vi "CODMn通讯.vi"() -> ()   [LabVIEW 2016, in "斯坦道CODMn新电路板.lvlib"]
uses:
  <vilib>/NI/Modbus Library/API/Wrapper/Create TCP Slave.vi
  <vilib>/Utility/config.llb/Write Key (String).vi
  <vilib>/Plasmionique/MB Master/MB_Master/MB_Master.lvclass
  <vilib>/NI/Modbus Library/API/slave/Modbus Slave.lvclass
  <vilib>/Utility/config.llb/NI_LVConfig.lvlib
  <vilib>/Plasmionique/MB Master/MB Master.lvlib
  <vilib>/NI/Modbus Library/API/Wrapper/API Main.lvlib
panel:
  out "控制命令 2":u16[](array[numeric]) format="%xH"
  out "状态告警区":T1 {"工作状态" items=["空闲"=0, "水样测试"=1, "标样核查"=2, "零点核查"=3, "跨度核查"=4, "空白测试"=5, "平行样测试"=6, "加标回收"=7, "空白校准"=8, "标样校准"=9, "初始化（清洗）"=10, "调试"=22, "填充管路"=30, "清洗管路"=31, "清洗反应杯"=32]; "告警代码" items=["无告警", "缺试剂告警", "缺水样告警", "缺蒸馏水告警", "缺标液告警", "仪表漏液告警", "标定异常告警", "超量程告警", "加热异常", "低试剂预警", "超上限告警", "超下限告警", "仪表内部其他异常", "滴定异常告警", "电极异常告警", "量程切换告警", "参数设置告警", "PH电极电位异常", "电导率电极异常", "浊度光度异常", "溶解氧电极异常", "溶解氧光强异常", "温度异常告警", "PH异常告警", "溶解氧异常告警", "电导率异常告警", "浊度异常告警", "叶绿素异常告警", "藻密度异常告警", "蓝绿藻异常告警", "ORP异常告警", "氨氮异常告警", "清洁刷异常告警", "SD卡异常告警", "蓝牙异常告警", "Wifi异常告警", "流程异常告警"]; "故障代码" items=["无故障", "电机故障", "温度故障", "通讯故障", "滴定故障"]}
  out "测量数据区":T2 {"单位" items=["ug/L", "mg/L", "ppm", "mg/m3", "cm", "ppb", "ug/m3", "%", "nmol/mol", "umol/mol", "MPN/L", "MPN/100ml", "ng/m3", "NTU", "无量纲", "ms/cm", "us/cm", "℃", "mV", "万个/L"]}
  out "状态告警区":u16[](array[numeric])
  out "测量数据区":u16[](array[numeric])
  out "序列号":string
  out "status":bool
  out "关键参数区":T3
  in  "读关键参数区":bool
  in  "读状态告警区":bool
  in  "读测量数据区":bool
  in  "站号":u16(ring) items=["CODMn"=21, "氨氮"=3]
  in  "停止":bool
  in  "启动":bool
  in  "控制命令":u16(ring) items=["启动测量"=1, "标样核查"=2, "零点核查"=3, "跨度核查"=4, "空白测试"=5, "平行样测试"=6, "加标回收"=7, "空白校准"=8, "标样校准"=9, "初始化（清洗）"=10, "停止测试"=11, "仪器重启"=12, "校时"=13, "模式设置"=14, "测量间隔设置"=15]
  in  "控制命令参数":u16[](array[numeric]) format="%04xH"
  in  "VISA Resource":refnum<visa-resource-name>
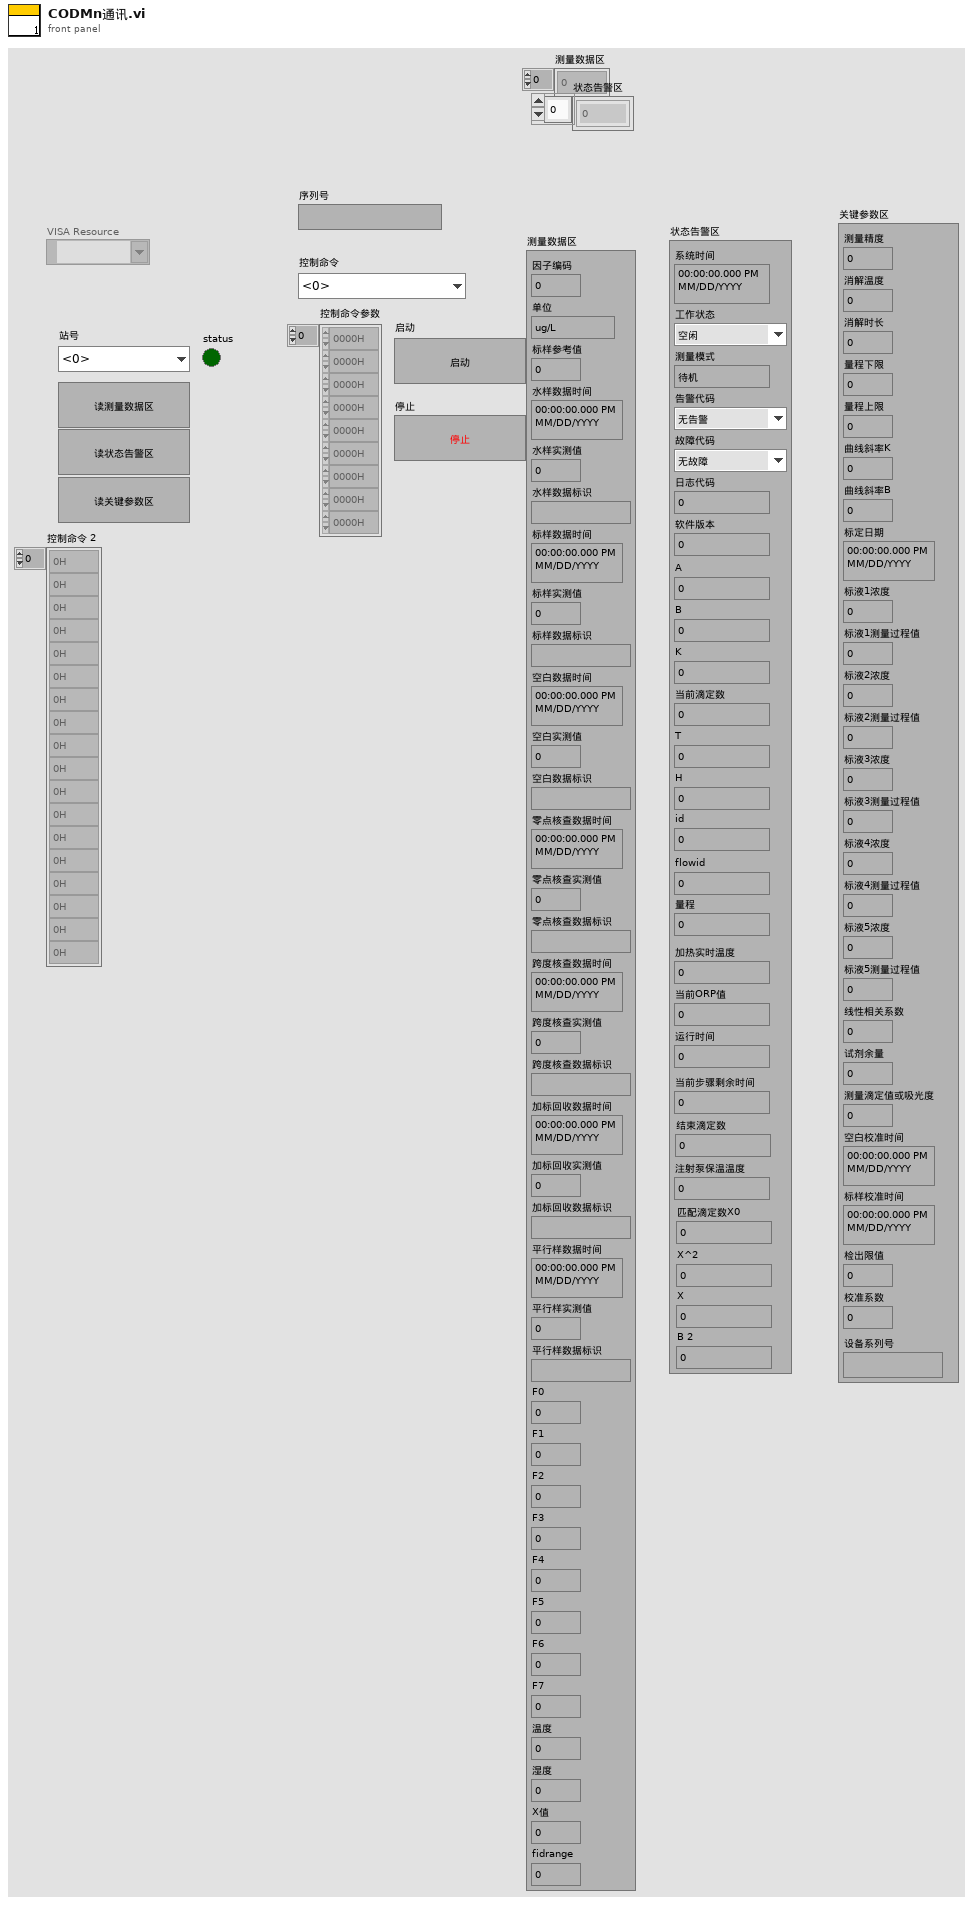
[diagram p1: front panel]
types:
  T1 = cluster{"系统时间":timestamp, "工作状态":u16, "测量模式":enum16{"待机", "连续模式", "周期模式", "定点模式", "受控模式", "手动模式"}, "告警代码":u16, "故障代码":u16, "日志代码":u16, "软件版本":u16, "A":sgl, "B":sgl, "K":sgl, "当前滴定数":sgl, "T":sgl, "H":sgl, "id":u16, "flowid":u16, "量程":u16, "加热实时温度":sgl, "当前ORP值":sgl, "运行时间":sgl, "当前步骤剩余时间":sgl, "结束滴定数":sgl, "注射泵保温温度":sgl, "匹配滴定数X0":u16, "X^2":sgl, "X":sgl, "B 2":sgl}
  T2 = cluster{"因子编码":u32, "单位":u16, "标样参考值":sgl, "水样数据时间":timestamp, "水样实测值":sgl, "水样数据标识":string, "标样数据时间":timestamp, "标样实测值":sgl, "标样数据标识":string, "空白数据时间":timestamp, "空白实测值":sgl, "空白数据标识":string, "零点核查数据时间":timestamp, "零点核查实测值":sgl, "零点核查数据标识":string, "跨度核查数据时间":timestamp, "跨度核查实测值":sgl, "跨度核查数据标识":string, "加标回收数据时间":timestamp, "加标回收实测值":sgl, "加标回收数据标识":string, "平行样数据时间":timestamp, "平行样实测值":sgl, "平行样数据标识":string, "F0":sgl, "F1":sgl, "F2":sgl, "F3":sgl, "F4":sgl, "F5":sgl, "F6":sgl, "F7":sgl, "温度":sgl, "湿度":sgl, "X值":sgl, "fidrange":sgl}
  T3 = cluster{"测量精度":u16, "消解温度":u16, "消解时长":u16, "量程下限":sgl, "量程上限":sgl, "曲线斜率K":sgl, "曲线斜率B":sgl, "标定日期":timestamp, "标液1浓度":sgl, "标液1测量过程值":sgl, "标液2浓度":sgl, "标液2测量过程值":sgl, "标液3浓度":sgl, "标液3测量过程值":sgl, "标液4浓度":sgl, "标液4测量过程值":sgl, "标液5浓度":sgl, "标液5测量过程值":sgl, "线性相关系数":sgl, "试剂余量":u32, "测量滴定值或吸光度":sgl, "空白校准时间":timestamp, "标样校准时间":timestamp, "检出限值":sgl, "校准系数":sgl, "设备系列号":string}
  T4 = cluster{"测量模式":enum16{"水样测量", "标样核查", "零点核查", "跨度核查", "空白测试", "加标回收", "平行样", "校零", "校标"}}
  T5 = typedef "NI_LVConfig.lvlib/Config Data RefNum.ctl" = refnum<k1>
  T6 = cluster{"站号":u16, "量程切换":enum32{"H", "L", "AUTO"}, "控制命令":u16, "模式设置":enum16{"待机", "连续模式", "周期模式", "定点模式", "受控模式", "手动模式"}, "测量间隔":u16}
  T7 = enum16{"水样测量", "标样核查", "零点核查", "跨度核查", "空白测试", "加标回收", "平行样", "校零", "校标"}
  T8 = enum8{"Enabled", "Disabled", "Disabled and Grayed Out"}
  T9 = typedef "量程选择控件.ctl" = enum32{"L", "H", "AUTO"}
  T10 = cluster{"水样测试量程模式":T9, "标样核查量程模式":T9, "零点核查量程模式":T9, "跨度核查量程模式":T9, "空白测试量程模式":T9, "平行样测试量程模式":T9, "加标回收量程模式":T9, "空白校准量程模式":T9, "标样校准量程模式":T9}
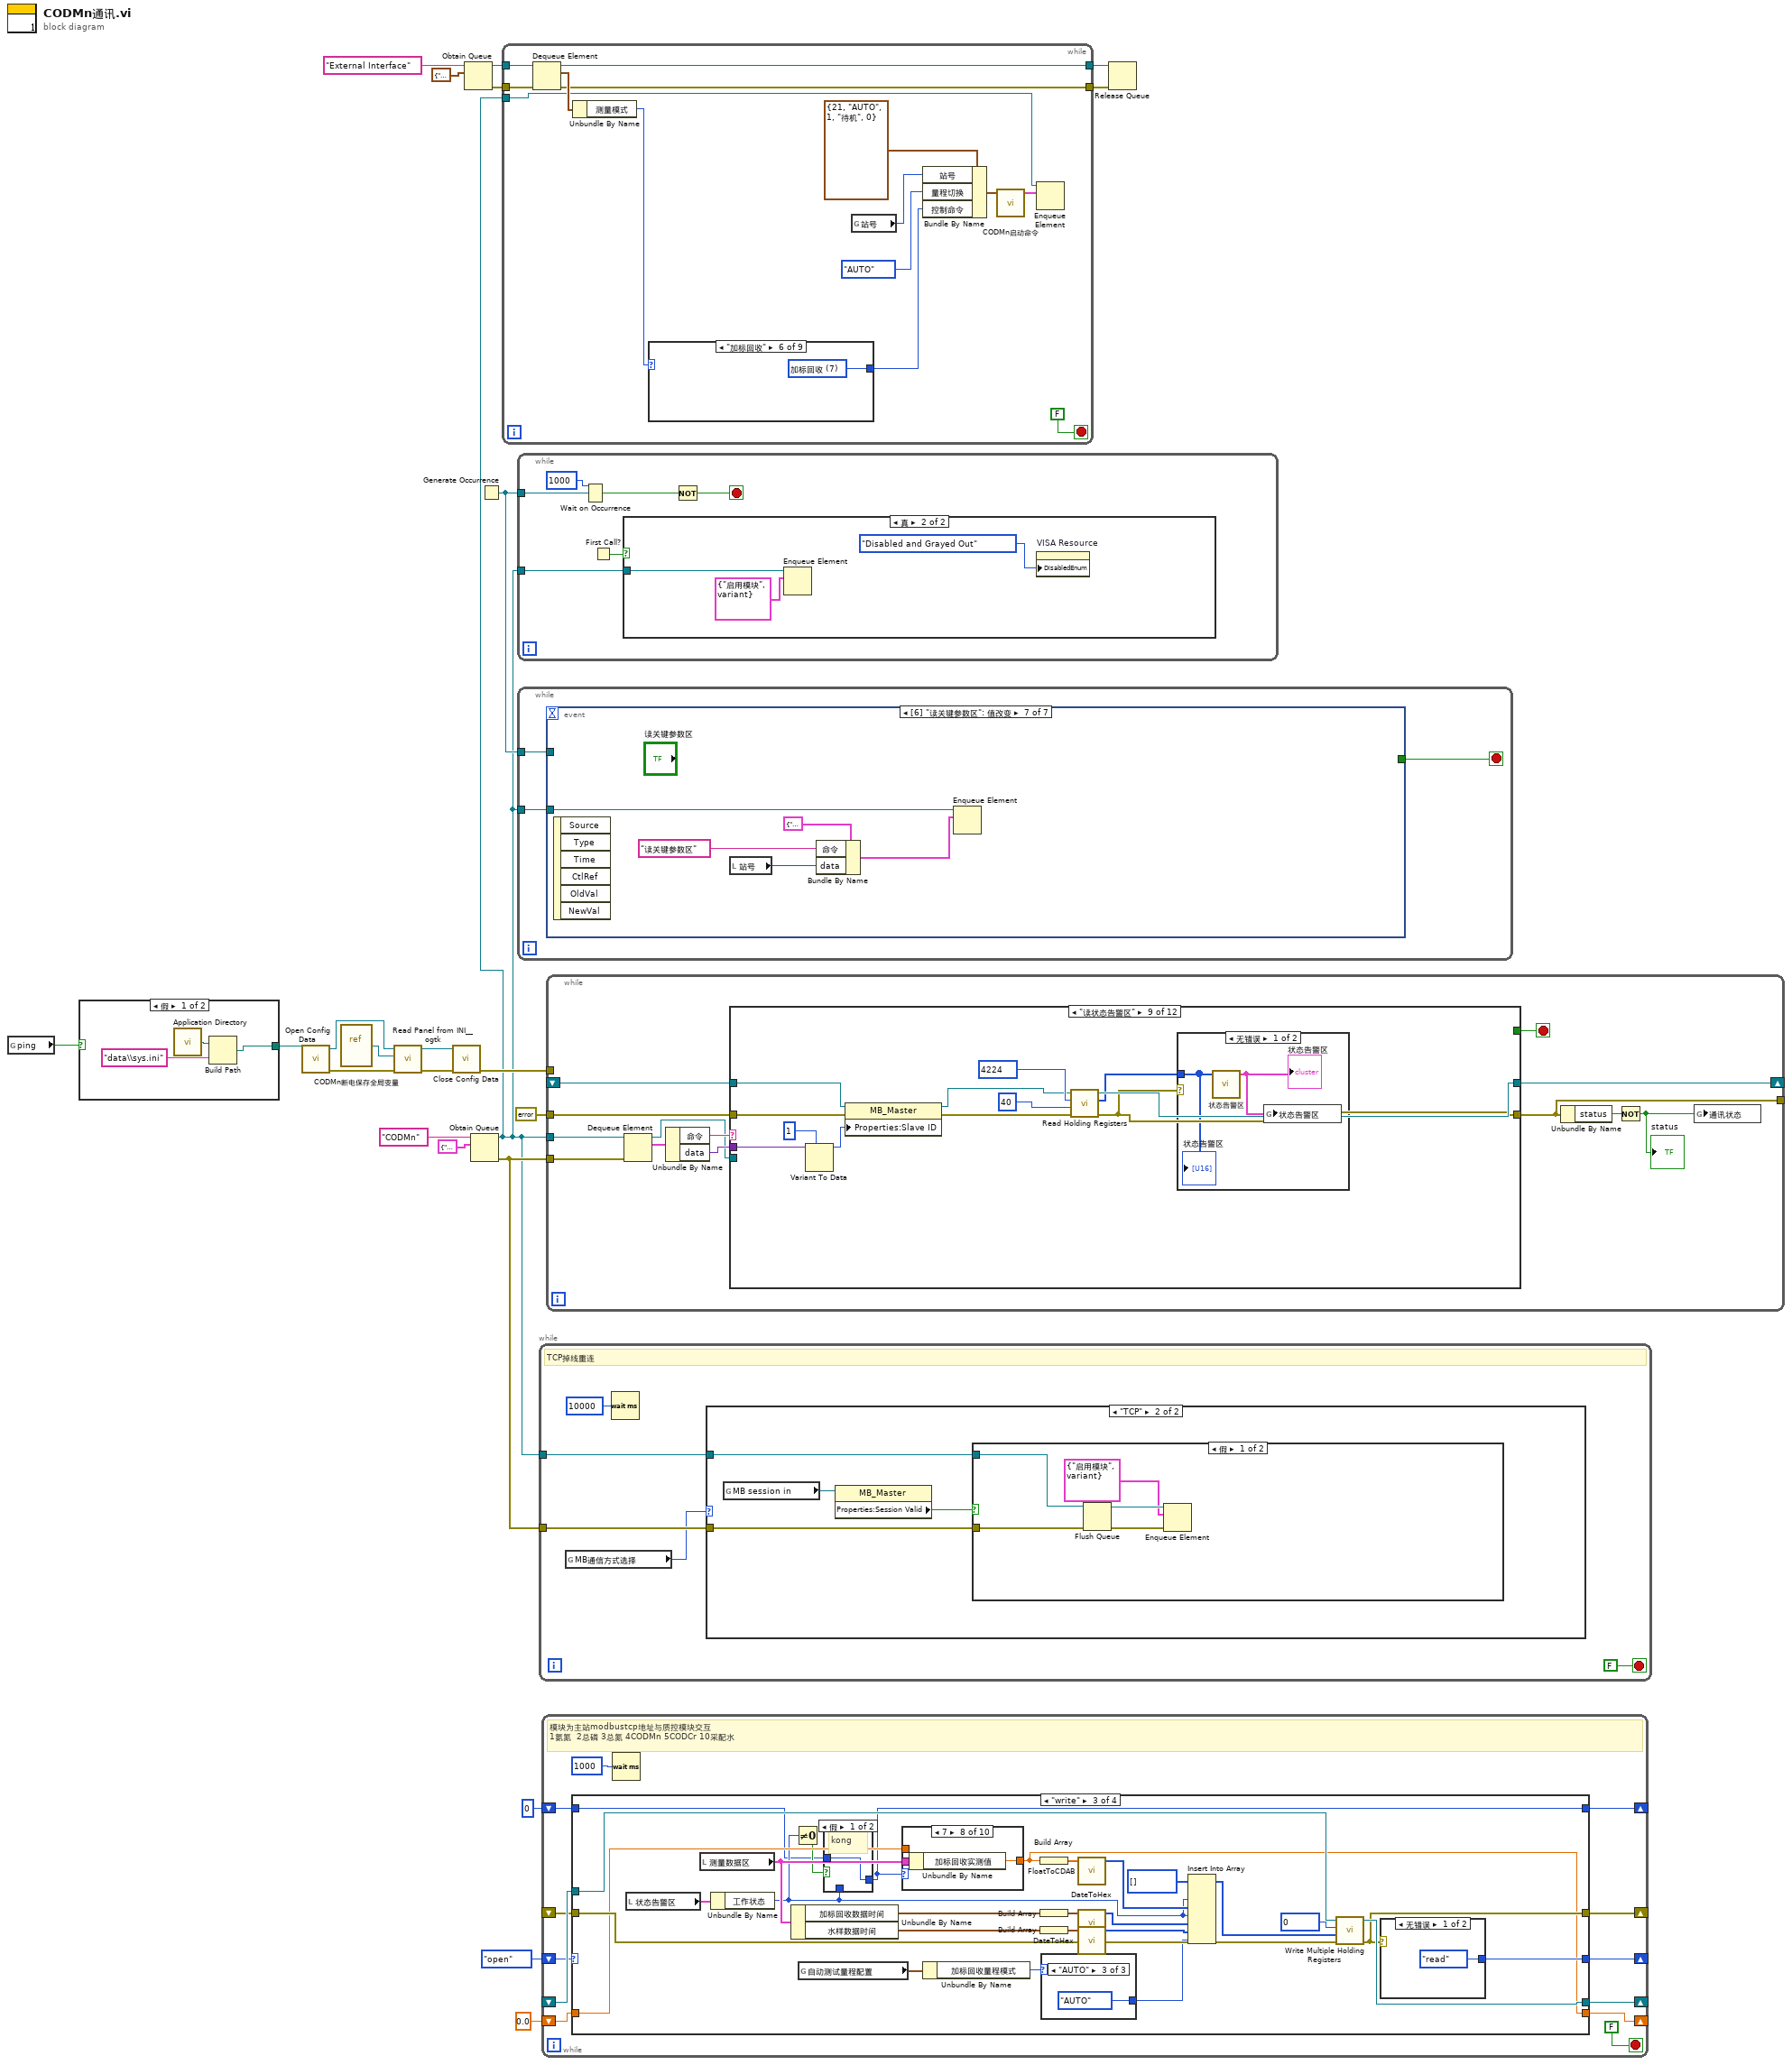
[diagram p0: block diagram]
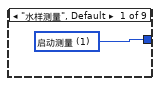
[diagram p2: hidden frame]
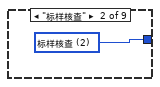
[diagram p3: hidden frame]
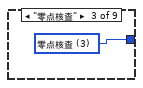
[diagram p4: hidden frame]
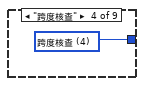
[diagram p5: hidden frame]
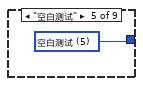
[diagram p6: hidden frame]
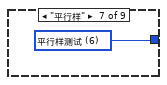
[diagram p7: hidden frame]
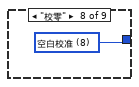
[diagram p8: hidden frame]
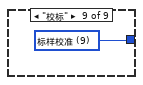
[diagram p9: hidden frame]
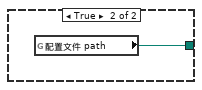
[diagram p10: hidden frame]
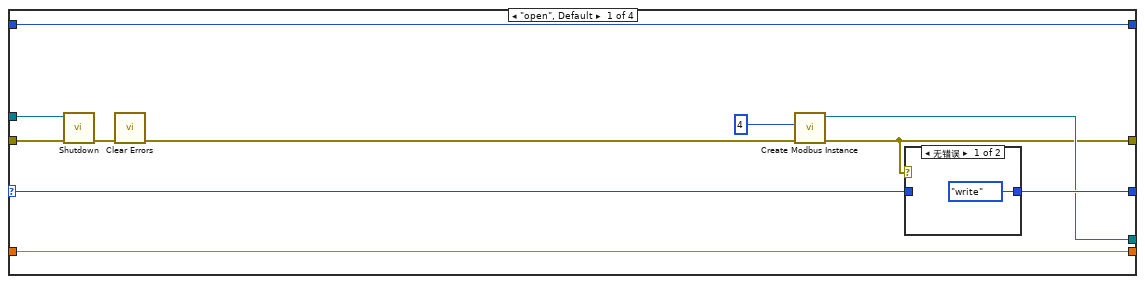
[diagram p13: hidden frame]
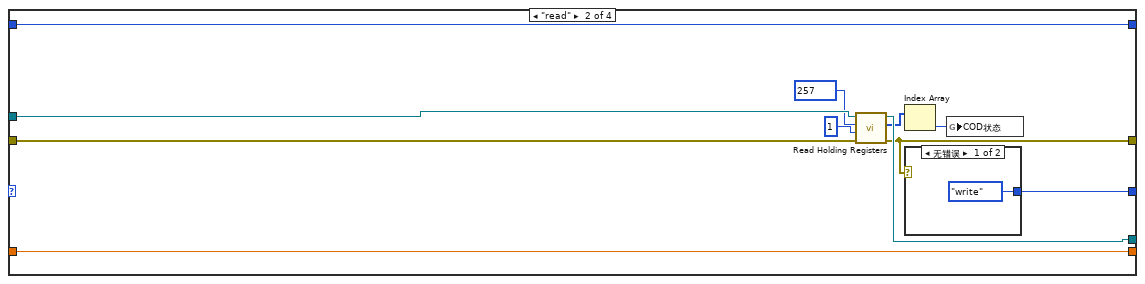
[diagram p15: hidden frame]
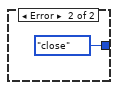
[diagram p16: hidden frame]
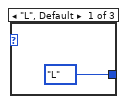
[diagram p17: hidden frame]
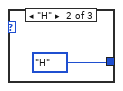
[diagram p18: hidden frame]
diagram:
  n1 = global read "VARCODMn全局变量.vi" "ping"() -> (w11:bool)
  n2 = case shown="假" w11 {
    tunnel: [w24 w27] -> w10
    frame False {
      n3 = call <vilib>:"Application Directory.vi"() -> ("Application Directory"=w26:path)
      n4 = Build Path(base path=w26, name or relative path="data\\sys.ini" ("名称或相对路径")) -> (appended path=w24:path)
    }
    frame True {
      n5 = global read "VARCODMn全局变量.vi" "配置文件 path"() -> (w27:path)
    }
  }
  n6 = call <vilib>:"Open Config Data.vi"("configuration file path"=w10) -> ("error out"=w18:errorcluster, "refnum"=w15:T5)  [unwired: 8 in, 1 out]
  n7 = vi-ref "CODMn断电保存全局变量.vi"() -> (w16:refnum<vi>)
  n8 = call <userlib>:"Read Panel from INI__ogtk.vi"("error in (no error)"=w18, "VI ref"=w16, "refnum"=w15) -> ("error out"=w19:errorcluster, "refnum out"=w17:T5)  [unwired: 7 in]
  n9 = call <vilib>:"Close Config Data.vi"("error in (no error)"=w19, "refnum"=w17) -> ("error out"=w14:errorcluster)  [unwired: 8 in, 1 out]
  n10 = Obtain Queue(name (unnamed)="External Interface" ("名称（未命名）"), element data type=T4 {"测量模式"=enum."水样测量"} ("元素")) -> (queue out=w7:refnum<queue>, error out=w6:errorcluster)  [unwired: 3 in, 1 out]
  n11 = Obtain Queue(name (unnamed)="CODMn" ("名称（未命名）"), element data type=cluster{"命令":string, "data":variant} {"命令"="", "data"=variant}) -> (queue out=w5:refnum<queue>, error out=w12:errorcluster)  [unwired: 3 in, 1 out]
  n12 = Generate Occurrence() -> (w20:refnum<k4>)
  n13 = while {
    tunnel: w7 -> [w41]
    tunnel: w6 -> [w40]
    tunnel: w5 -> [w32]
    tunnel: [w31] -> w4
    tunnel: [w30] -> w3
    stop <- FALSE stop-if-true
    n14 = Dequeue Element(queue=w41, error in (no error)=w40) -> (queue out=w31:refnum<queue>, element=w35:T4, error out=w30:errorcluster)  [unwired: 1 in, 1 out]
    n15 = Unbundle By Name(w35) -> ("测量模式"=w34:T7)
    n16 = case shown="\"加标回收\"" w34 {
      tunnel: [w42 w43 w44 w45 w46 w47 w48 w49 w50] -> w33
      frame "水样测量", Default {
        w42 = u16 1 items=["启动测量"=1, "标样核查"=2, "零点核查"=3, "跨度核查"=4, "空白测试"=5, "平行样测试"=6, "加标回收"=7, "空白校准"=8, "标样校准"=9, "初始化（清洗）"=10, "停止测试"=11, "仪器重启"=12, "校时"=13, "模式设置"=14, "测量间隔设置"=15, "调试"=22, "填充管路"=30, "清洗管路"=31, "清洗反应杯"=32] ("控制命令")
      }
      frame "标样核查" {
        w43 = u16 2 items=["启动测量"=1, "标样核查"=2, "零点核查"=3, "跨度核查"=4, "空白测试"=5, "平行样测试"=6, "加标回收"=7, "空白校准"=8, "标样校准"=9, "初始化（清洗）"=10, "停止测试"=11, "仪器重启"=12, "校时"=13, "模式设置"=14, "测量间隔设置"=15, "调试"=22, "填充管路"=30, "清洗管路"=31, "清洗反应杯"=32] ("控制命令")
      }
      frame "零点核查" {
        w44 = u16 3 items=["启动测量"=1, "标样核查"=2, "零点核查"=3, "跨度核查"=4, "空白测试"=5, "平行样测试"=6, "加标回收"=7, "空白校准"=8, "标样校准"=9, "初始化（清洗）"=10, "停止测试"=11, "仪器重启"=12, "校时"=13, "模式设置"=14, "测量间隔设置"=15, "调试"=22, "填充管路"=30, "清洗管路"=31, "清洗反应杯"=32] ("控制命令")
      }
      frame "跨度核查" {
        w45 = u16 4 items=["启动测量"=1, "标样核查"=2, "零点核查"=3, "跨度核查"=4, "空白测试"=5, "平行样测试"=6, "加标回收"=7, "空白校准"=8, "标样校准"=9, "初始化（清洗）"=10, "停止测试"=11, "仪器重启"=12, "校时"=13, "模式设置"=14, "测量间隔设置"=15, "调试"=22, "填充管路"=30, "清洗管路"=31, "清洗反应杯"=32] ("控制命令")
      }
      frame "空白测试" {
        w46 = u16 5 items=["启动测量"=1, "标样核查"=2, "零点核查"=3, "跨度核查"=4, "空白测试"=5, "平行样测试"=6, "加标回收"=7, "空白校准"=8, "标样校准"=9, "初始化（清洗）"=10, "停止测试"=11, "仪器重启"=12, "校时"=13, "模式设置"=14, "测量间隔设置"=15, "调试"=22, "填充管路"=30, "清洗管路"=31, "清洗反应杯"=32] ("控制命令")
      }
      frame "加标回收" {
        w47 = u16 7 items=["启动测量"=1, "标样核查"=2, "零点核查"=3, "跨度核查"=4, "空白测试"=5, "平行样测试"=6, "加标回收"=7, "空白校准"=8, "标样校准"=9, "初始化（清洗）"=10, "停止测试"=11, "仪器重启"=12, "校时"=13, "模式设置"=14, "测量间隔设置"=15, "调试"=22, "填充管路"=30, "清洗管路"=31, "清洗反应杯"=32] ("控制命令")
      }
      frame "平行样" {
        w48 = u16 6 items=["启动测量"=1, "标样核查"=2, "零点核查"=3, "跨度核查"=4, "空白测试"=5, "平行样测试"=6, "加标回收"=7, "空白校准"=8, "标样校准"=9, "初始化（清洗）"=10, "停止测试"=11, "仪器重启"=12, "校时"=13, "模式设置"=14, "测量间隔设置"=15, "调试"=22, "填充管路"=30, "清洗管路"=31, "清洗反应杯"=32] ("控制命令")
      }
      frame "校零" {
        w49 = u16 8 items=["启动测量"=1, "标样核查"=2, "零点核查"=3, "跨度核查"=4, "空白测试"=5, "平行样测试"=6, "加标回收"=7, "空白校准"=8, "标样校准"=9, "初始化（清洗）"=10, "停止测试"=11, "仪器重启"=12, "校时"=13, "模式设置"=14, "测量间隔设置"=15, "调试"=22, "填充管路"=30, "清洗管路"=31, "清洗反应杯"=32] ("控制命令")
      }
      frame "校标" {
        w50 = u16 9 items=["启动测量"=1, "标样核查"=2, "零点核查"=3, "跨度核查"=4, "空白测试"=5, "平行样测试"=6, "加标回收"=7, "空白校准"=8, "标样校准"=9, "初始化（清洗）"=10, "停止测试"=11, "仪器重启"=12, "校时"=13, "模式设置"=14, "测量间隔设置"=15, "调试"=22, "填充管路"=30, "清洗管路"=31, "清洗反应杯"=32] ("控制命令")
      }
    }
    n17 = global read "CODMn断电保存全局变量.vi" "站号"() -> (w36:u16)
    n18 = Bundle By Name(cluster=T6 {"站号"=21, "量程切换"=enum."AUTO", "控制命令"=1, "模式设置"=enum."待机", "测量间隔"=0} ("参数"), "站号"=w36, "量程切换"=enum32{"H", "L", "AUTO"}."AUTO", "控制命令"=w33) -> (w37:T6)
    n19 = call "CODMn启动命令.vi"("参数"=w37) -> ("启动命令"=w39:cluster{"命令":string, "data":variant})  [unwired: 10 in]
    n20 = Enqueue Element(queue=w32, element=w39) -> ()  [unwired: 2 in, 3 out]
  }
  n21 = while {
    tunnel: w20 -> [w56]
    tunnel: w5 -> [w52]
    stop <- w53 stop-if-true
    n22 = Wait on Occurrence(2:w56, 3:1000 ("毫秒超时(-1)")) -> (0:w54:bool)  [unwired: 1 in]
    n23 = First Call?() -> (First Call?: T/F=w51:bool)
    n24 = case shown="真" w51 {
      tunnel: w52 -> [_ w58]
      frame False {
      }
      frame True {
        n25 = Enqueue Element(queue=w58, element=cluster{"命令":string, "data":variant} {"命令"="启用模块", "data"=variant} ("元素")) -> ()  [unwired: 2 in, 3 out]
        n26 = property on="VISA Resource" class="VISAName"("DisabledEnum"=T8."Disabled and Grayed Out" ("禁用")) -> ()  [unwired: 2 in, 2 out]
      }
    }
    n27 = Not(x=w54) -> (.not. x?=w53:bool)
  }
  n28 = while {
    tunnel: w5 -> [w62]
    tunnel: w20 -> [w60]
    stop <- w61 stop-if-true
    n29 = event shown="[6] \"读关键参数区\": 值改变" {
      selector: _ -> [_ _ _ _ _ _ _]
      dyn-events: _ -> [_ _ _ _ _ _ _]
      timeout: _ -> [_ _ _ _ _ _ _]
      tunnel: w62 -> [_ _ w83 w90 w96 w101 w106]
      tunnel: [_ _ _ "停止" _ _ _] -> w61
      tunnel: w60 -> [_ _ _ w87 _ _ _]
      event Timeout {
        n30 = event-data() -> ()  [unwired: 1 in, 3 out]
      }
      event "VISA Resource": Value Change {
        n31 = event-data() -> ()  [unwired: 1 in, 6 out]
        n32 = call <vilib>:"Application Directory.vi"() -> ("Application Directory"=w65:path)
        n33 = Build Path(base path=w65, name or relative path="data\\set.ini" ("名称或相对路径")) -> (appended path=w66:path)
        n34 = call <vilib>:"Open Config Data.vi"("configuration file path"=w66) -> ("error out"=w72:errorcluster, "refnum"=w71:T5)  [unwired: 8 in, 1 out]
        n35 = call-poly <vilib>:"Write Key.vi"("section"="CODMn", "error in (no error)"=w72, "value"="VISA Resource", "key"="串口", "refnum"=w71) -> ("error out"=w68:errorcluster, "refnum out"=w64:T5)  [unwired: 4 in, 1 out]
        n36 = call <vilib>:"Close Config Data.vi"("error in (no error)"=w68, "refnum"=w64) -> ()  [unwired: 8 in, 2 out]
      }
      event "启动": Value Change {
        n37 = event-data() -> ()  [unwired: 1 in, 6 out]
        n38 = case shown="默认" "控制命令" {
          tunnel: "控制命令参数" -> [w85 w86]
          tunnel: [w84 w86] -> w73
          frame Default {
            n39 = call "HexToWord.vi"("数组"=w85) -> ("WORD"=w84:u16[])  [unwired: 10 in]
          }
          frame 13 {
          }
        }
        n40 = Swap Bytes(anything="控制命令") -> (byte swapped=w76:u16)
        n41 = call "控制命令区.vi"("控制命令参数"=w73, "控制命令"=w76) -> ("控制命令"=w79:u16[])  [unwired: 9 in]
        n42 = local read "站号"() -> (w78:u16)
        n43 = Bundle("站号"=w78, "控制命令"=w79) -> (w77:cluster{"站号":u16, "控制命令":u16[]})  [unwired: 1 in]
        n44 = Bundle By Name(cluster=cluster{"命令":string, "data":variant} {"命令"="", "data"=variant} ("元素"), "命令"="启动", "data"=w77) -> (w81:cluster{"命令":string, "data":variant})
        n45 = Enqueue Element(queue=w83, element=w81) -> ()  [unwired: 2 in, 3 out]
      }
      event "停止": Value Change {
        n46 = event-data() -> ()  [unwired: 1 in, 6 out]
        n47 = Set Occurrence(w87) -> ()
        n48 = Flush Queue(queue=w90) -> (queue out=w89:refnum<queue>)  [unwired: 1 in, 2 out]
        n49 = Enqueue Element(queue=w89, element=cluster{"命令":string, "data":variant} {"命令"="shutdown", "data"=variant} ("元素")) -> ()  [unwired: 2 in, 3 out]
      }
      event "读测量数据区": Value Change {
        n50 = event-data() -> ()  [unwired: 1 in, 6 out]
        n51 = Bundle By Name(cluster=cluster{"命令":string, "data":variant} {"命令"="", "data"=variant} ("元素"), "命令"="读测量数据区", "data"="站号") -> (w94:cluster{"命令":string, "data":variant})
        n52 = Enqueue Element(queue=w96, element=w94) -> ()  [unwired: 2 in, 3 out]
      }
      event "读状态告警区": Value Change {
        n53 = event-data() -> ()  [unwired: 1 in, 6 out]
        n54 = local read "站号"() -> (w97:u16)
        n55 = Bundle By Name(cluster=cluster{"命令":string, "data":variant} {"命令"="", "data"=variant} ("元素"), "命令"="读状态告警区", "data"=w97) -> (w99:cluster{"命令":string, "data":variant})
        n56 = Enqueue Element(queue=w101, element=w99) -> ()  [unwired: 2 in, 3 out]
      }
      event "读关键参数区": Value Change {
        n57 = event-data() -> ()  [unwired: 1 in, 6 out]
        n58 = local read "站号"() -> (w102:u16)
        n59 = Bundle By Name(cluster=cluster{"命令":string, "data":variant} {"命令"="", "data"=variant} ("元素"), "命令"="读关键参数区", "data"=w102) -> (w104:cluster{"命令":string, "data":variant})
        n60 = Enqueue Element(queue=w106, element=w104) -> ()  [unwired: 2 in, 3 out]
      }
    }
  }
  n61 = while "While循环" {
    tunnel: w5 -> [w109]
    tunnel: w12 -> [w108]
    stop <- FALSE stop-if-true
    # "TCP掉线重连"
    n62 = global read "CODMn断电保存全局变量.vi" "MB通信方式选择"() -> (w107:enum16{"串口", "TCP"})
    n63 = Wait (ms)(milliseconds to wait=u32 10000 ("等待时间（毫秒）")) -> ()  [unwired: 1 out]
    n64 = case shown="\"TCP\"" w107 {
      tunnel: w109 -> [_ w114]
      tunnel: w108 -> [_ w113]
      frame "串口", Default {
      }
      frame "TCP" {
        n65 = global read "VARCODMn全局变量.vi" "MB session in"() -> (w112:refnum<class "MB_Master.lvclass">)
        n66 = property class="MB_Master"(reference=w112) -> ("Properties:Session Valid"=w115:bool)  [unwired: 1 in, 2 out]
        n67 = case shown="假" w115 {
          tunnel: w114 -> [w118 _]
          tunnel: w113 -> [w117 _]
          frame False {
            n68 = Flush Queue(queue=w118, error in (no error)=w117) -> (queue out=w120:refnum<queue>, error out=w119:errorcluster)  [unwired: 1 out]
            n69 = Enqueue Element(queue=w120, element=cluster{"命令":string, "data":variant} {"命令"="启用模块", "data"=variant} ("元素"), error in (no error)=w119) -> ()  [unwired: 1 in, 3 out]
          }
          frame True {
          }
        }
      }
    }
  }
  n70 = while {
    shift-right: [w130] -> _
    shift-left: _ -> [w132]
    shift-right: [w129] -> _
    shift-left: _ -> [w131]
    shift-right: [w126] -> _
    shift-left: enum16{"open", "read", "write", "close"}."open" -> [w127]
    shift-right: [w124] -> _
    shift-left: sgl 0.0 ("标样实测值") -> [w123]
    shift-right: [w122] -> _
    shift-left: u16 0 ("工作状态") -> [w121]
    stop <- FALSE stop-if-true
    # "模块为主站modbustcp地址与质控模块交互\n1氨氮  2总磷 3总氮 4CODMn 5CODCr 10采配水"
    n71 = case shown="\"write\"" w127 {
      selector: w127 -> [w143 _ _ _]
      tunnel: w132 -> [w137 w155 w184 w216]
      tunnel: w131 -> [w136 w153 w183 w215]
      tunnel: [w140 w154 w181 w216] -> w130
      tunnel: [w139 w152 w180 w218] -> w129
      tunnel: [w142 w156 w185 enum16{"open", "read", "write", "close"}."open"] -> w126
      tunnel: [w134 w147 w175 w213] -> w124
      tunnel: w123 -> [w134 w147 w176 w213]
      tunnel: [w133 w146 w163 w212] -> w122
      tunnel: w121 -> [w133 w146 w162 w212]
      frame "open", Default {
        n72 = call-dynamic "Shutdown.vi"("error in"=w136, "Modbus slave in"=w137) -> ("error out"=w135:errorcluster)  [unwired: 9 in]
        n73 = call <vilib>:"Clear Errors.vi"("error in (no error)"=w135) -> ("error out"=w138:errorcluster)  [unwired: 5 in, 1 out]
        n74 = call-poly <vilib>:"Create Modbus Instance.vi"("error in"=w138, "port (502)"=u16 4) -> ("error out"=w139:errorcluster, "TCP slave instance"=w140:refnum<class "Modbus Slave.lvclass">)  [unwired: 8 in]
        n75 = case shown="无错误" w139 {
          tunnel: w143 -> [_ w145]
          tunnel: [enum16{"open", "read", "write", "close"}."write" w145] -> w142
          frame No Error {
          }
          frame Error {
          }
        }
      }
      frame "read" {
        n76 = call-dynamic <vilib>:"Read Holding Registers.vi"("error in"=w153, "number of inputs"=u16 1, "starting address"=u16 257, "Modbus slave in"=w155) -> ("error out"=w152:errorcluster, "register values"=w149:u16[], "Modbus slave out"=w154:refnum<class "Modbus Slave.lvclass">)  [unwired: 5 in]
        n77 = Index Array(array=w149) -> (element=w148:u16)  [unwired: 1 in]
        n78 = case shown="无错误" w152 {
          tunnel: [enum16{"open", "read", "write", "close"}."write" enum16{"open", "read", "write", "close"}."close"] -> w156
          frame No Error {
          }
          frame Error {
          }
        }
        n79 = global write "VARCODMn全局变量.vi" "COD状态"(w148) -> ()
      }
      frame "write" {
        n80 = local read "状态告警区"() -> (w177:T1)
        n81 = local read "测量数据区"() -> (w172:T2)
        n82 = Unbundle By Name(w177) -> ("工作状态"=w164:u16)
        n83 = Unbundle By Name(w172) -> ("加标回收数据时间"=w171:timestamp, "水样数据时间"=w168:timestamp)
        n84 = Not Equal To 0?(x=w164) -> (x != 0?=w165:bool)
        n85 = global read "CODMn断电保存全局变量.vi" "自动测试量程配置"() -> (w161:T10)
        n86 = case shown="假" w165 {
          tunnel: w164 -> [_ w190]
          tunnel: [w189 w190] -> w163
          tunnel: w162 -> [w189 _]
          frame False {
            # "kong"
          }
          frame True {
            # "..."
          }
        }
        n87 = case shown="7" w163 {
          tunnel: [w191 w193 w195 w197 w199 w201 w203 w205 w207 w209] -> w175
          tunnel: w176 -> [w191 _ _ _ _ _ _ _ _ _]
          tunnel: w172 -> [_ w192 w194 w196 w198 w200 w202 w204 w206 w208]
          frame 0, Default {
          }
          frame 1 {
            n88 = Unbundle By Name(w192) -> ("水样实测值"=w193:sgl)
          }
          frame 2 {
            n89 = Unbundle By Name(w194) -> ("标样实测值"=w195:sgl)
          }
          frame 3 {
            n90 = Unbundle By Name(w196) -> ("零点核查实测值"=w197:sgl)
          }
          frame 4 {
            n91 = Unbundle By Name(w198) -> ("跨度核查实测值"=w199:sgl)
          }
          frame 5 {
            n92 = Unbundle By Name(w200) -> ("空白实测值"=w201:sgl)
          }
          frame 6 {
            n93 = Unbundle By Name(w202) -> ("平行样实测值"=w203:sgl)
          }
          frame 7 {
            n94 = Unbundle By Name(w204) -> ("加标回收实测值"=w205:sgl)
          }
          frame 8 {
            n95 = Unbundle By Name(w206) -> ("空白实测值"=w207:sgl)
          }
          frame 9 {
            n96 = Unbundle By Name(w208) -> ("标样实测值"=w209:sgl)
          }
        }
        n97 = Unbundle By Name(w161) -> ("加标回收量程模式"=w160:T9)
        n98 = Build Array(w175) -> (w174:sgl[])
        n99 = Build Array(w171) -> (w170:timestamp[])
        n100 = Build Array(w168) -> (w167:timestamp[])
        n101 = case shown="\"AUTO\"" w160 {
          tunnel: [enum32{"H", "L", "AUTO"}."L" ("加标回收量程选择") enum32{"H", "L", "AUTO"}."H" ("加标回收量程选择") enum32{"H", "L", "AUTO"}."AUTO" ("加标回收量程选择")] -> w159
          frame "L", Default {
          }
          frame "H" {
          }
          frame "AUTO" {
          }
        }
        n102 = call "FloatToCDAB.vi"("浮点数"=w174) -> ("CDAB整形输出"=w173:u16[])  [unwired: 10 in]
        n103 = call "DateToHex.vi"("DATE"=w170) -> ("数组"=w169:u16[])  [unwired: 10 in]
        n104 = call "DateToHex.vi"("DATE"=w167) -> ("数组"=w166:u16[])  [unwired: 10 in]
        n105 = Insert Into Array(array=u16[] [] ("values"), new element #1=w164, new element #2=w173, new element #3=w164, new element #4=w169, new element #5=w166, new element #6=w159) -> (w178:u16[])  [unwired: 1 in]
        n106 = call-dynamic "Write Multiple Holding Registers.vi"("error in"=w183, "registers to write"=w178, "starting address"=u16 0, "Modbus slave in"=w184) -> ("error out"=w180:errorcluster, "Modbus slave out"=w181:refnum<class "Modbus Slave.lvclass">)  [unwired: 6 in]
        n107 = case shown="无错误" w180 {
          tunnel: [enum16{"open", "read", "write", "close"}."read" enum16{"open", "read", "write", "close"}."close"] -> w185
          frame No Error {
          }
          frame Error {
          }
        }
      }
      frame "close" {
        n108 = call-dynamic "Shutdown.vi"("error in"=w215, "Modbus slave in"=w216) -> ("error out"=w214:errorcluster)  [unwired: 9 in]
        n109 = call <vilib>:"Clear Errors.vi"("error in (no error)"=w214) -> ("error out"=w218:errorcluster)  [unwired: 5 in, 1 out]
      }
    }
    n110 = Wait (ms)(milliseconds to wait=u32 1000 ("等待时间（毫秒）")) -> ()  [unwired: 1 out]
  }
  n111 = while {
    tunnel: w5 -> [w231]
    tunnel: w12 -> [w230]
    shift-right: [w228] -> _
    shift-left: _ -> [w227]
    tunnel: errorcluster {"status"=FALSE, "code"=0, "source"=""} ("error out") -> [w226]
    tunnel: [w221] -> _
    tunnel: w14 -> [_]
    stop <- w229 stop-if-true
    n112 = Dequeue Element(queue=w231, error in (no error)=w230) -> (queue out=w222:refnum<queue>, element=w224:cluster{"命令":string, "data":variant})  [unwired: 1 in, 2 out]
    n113 = Unbundle By Name(w224) -> ("命令"=w225:string, "data"=w223:variant)
    n114 = case shown="\"读状态告警区\"" w225 {
      tunnel: w223 -> [_ _ _ w250 w261 w278 w290 w299 w309 w325 w340 _]
      tunnel: w222 -> [_ _ _ _ _ _ _ _ _ _ _ w353]
      tunnel: [_ _ _ _ _ _ _ _ _ _ _ TRUE] -> w229
      tunnel: [w232 w235 w237 w253 w264 w280 w292 w304 w318 w332 w347 w349] -> w228
      tunnel: [w233 w234 w238 w252 w263 w279 w291 w293 w307 w321 w348 w350] -> w221
      tunnel: w227 -> [w232 _ w237 w249 w260 w277 w289 w298 w312 w328 w343 w349]
      tunnel: w226 -> [w233 _ w240 w246 w257 w274 w286 w296 w313 w329 w344 w351]
      frame Default {
      }
      frame "启用模块" {
        n115 = call "MB_api.vi"("STEP"=enum16{"open", "read", "write", "close"}."open") -> ("error out"=w234:errorcluster, "MB session out"=w235:refnum<class "MB_Master.lvclass">)  [unwired: 8 in, 1 out]
        n116 = global write "VARCODMn全局变量.vi" "MB session in"(w235) -> ()
      }
      frame "停用模块" {
        n117 = call-dynamic "Close Session.vi"("error in (no error)"=w240, "MB session in"=w237) -> ("error out"=w239:errorcluster)  [unwired: 9 in]
        n118 = call <vilib>:"Clear Errors.vi"("error in (no error)"=w239) -> ("error out"=w238:errorcluster)  [unwired: 5 in, 1 out]
      }
      frame "启动" {
        n119 = Variant To Data(type=cluster{"站号":u16, "控制命令":u16[]} {"站号"=0, "控制命令"=[]} ("输出簇"), Variant=w250) -> (data=w244:cluster{"站号":u16, "控制命令":u16[]})  [unwired: 1 in, 1 out]
        n120 = Unbundle By Name(w244) -> ("站号"=w243:u16, "控制命令"=w241:u16[])
        n121 = property class="MB_Master"(reference=w249, error in=w246, "Properties:Slave ID"=w243) -> (reference out=w248:refnum<class "MB_Master.lvclass">, error out=w247:errorcluster)
        n122 = Index Array(array=w241) -> (element=w242:u16)  [unwired: 1 in]
        n123 = global write "VARCODMn全局变量.vi" "控制命令"(w242) -> ()
        n124 = call <vilib>:"Write Multiple Registers.vi"("error in (no error)"=w247, "values"=w241, "starting address"=u16 4608, "MB session in"=w248) -> ("error out"=w252:errorcluster, "MB session out"=w253:refnum<class "MB_Master.lvclass">)  [unwired: 6 in]
      }
      frame "盲样测试" {
        n125 = Variant To Data(type=0, Variant=w261) -> (data=w254:i32)  [unwired: 1 in, 1 out]
        n126 = property class="MB_Master"(reference=w260, error in=w257, "Properties:Slave ID"=w254) -> (reference out=w259:refnum<class "MB_Master.lvclass">, error out=w258:errorcluster)
        n127 = case shown="默认" w254 {
          tunnel: [u16[] [] ("values") u16[] [33539, 0] ("values") u16[] [23555, 0] ("values")] -> w256
          frame Default {
          }
          frame 1 {
            # "总磷盲样测试命令"
          }
          frame 3 {
            # "氨氮盲样测试"
          }
        }
        n128 = call <vilib>:"Write Multiple Registers.vi"("error in (no error)"=w258, "values"=w256, "starting address"=u16 24592, "MB session in"=w259) -> ("error out"=w263:errorcluster, "MB session out"=w264:refnum<class "MB_Master.lvclass">)  [unwired: 6 in]
      }
      frame "debug" {
        n129 = Variant To Data(type=cluster{"站号":u16, "控制命令":u16[]} {"站号"=0, "控制命令"=[]} ("输出簇"), Variant=w278) -> (data=w272:cluster{"站号":u16, "控制命令":u16[]})  [unwired: 1 in, 1 out]
        n130 = Unbundle By Name(w272) -> ("站号"=w271:u16, "控制命令"=w269:u16[])
        "控制命令 2" <- w269
        n131 = property class="MB_Master"(reference=w277, error in=w274, "Properties:Slave ID"=w271) -> (reference out=w276:refnum<class "MB_Master.lvclass">, error out=w275:errorcluster)
        n132 = Index Array(array=w269) -> (element=w270:u16)  [unwired: 1 in]
        n133 = global write "VARCODMn全局变量.vi" "控制命令"(w270) -> ()
        n134 = call <vilib>:"Write Multiple Registers.vi"("error in (no error)"=w275, "values"=w269, "starting address"=u16 24594, "MB session in"=w276) -> ("error out"=w279:errorcluster, "MB session out"=w280:refnum<class "MB_Master.lvclass">)  [unwired: 6 in]
      }
      frame "单步控制" {
        n135 = Variant To Data(type=cluster{"站号":u16, "控制命令":u16[]} {"站号"=0, "控制命令"=[]} ("输出簇"), Variant=w290) -> (data=w284:cluster{"站号":u16, "控制命令":u16[]})  [unwired: 1 in, 1 out]
        n136 = Unbundle By Name(w284) -> ("站号"=w283:u16, "控制命令"=w282:u16[])
        n137 = property class="MB_Master"(reference=w289, error in=w286, "Properties:Slave ID"=w283) -> (reference out=w288:refnum<class "MB_Master.lvclass">, error out=w287:errorcluster)
        n138 = call <vilib>:"Write Multiple Registers.vi"("error in (no error)"=w287, "values"=w282, "starting address"=u16 24610, "MB session in"=w288) -> ("error out"=w291:errorcluster, "MB session out"=w292:refnum<class "MB_Master.lvclass">)  [unwired: 6 in]
      }
      frame "读测量数据区" {
        n139 = Variant To Data(type=u8 1 ("Slave ID"), Variant=w299) -> (data=w300:u8)  [unwired: 1 in, 1 out]
        n140 = property class="MB_Master"(reference=w298, error in=w296, "Properties:Slave ID"=w300) -> (reference out=w297:refnum<class "MB_Master.lvclass">, error out=w295:errorcluster)
        n141 = call <vilib>:"Read Holding Registers.vi"("error in (no error)"=w295, "quantity"=u16 105, "starting address"=u16 4096, "MB session in"=w297) -> ("error out"=w293:errorcluster, "Registers"=w294:u16[], "MB session out"=w304:refnum<class "MB_Master.lvclass">)  [unwired: 5 in]
        n142 = case shown="无错误" w293 {
          tunnel: w294 -> [w306 _]
          frame No Error {
            n143 = call "测量数据区.vi"("数组"=w306) -> ("测量数据区"=w305:T2)  [unwired: 10 in]
            "测量数据区" <- w305
            n144 = global write "VARCODMn全局变量.vi" "测量数据区"(w305) -> ()
            "测量数据区" <- w306
          }
          frame Error {
          }
        }
      }
      frame "读状态告警区" {
        n145 = Variant To Data(type=u8 1 ("Slave ID"), Variant=w309) -> (data=w314:u8)  [unwired: 1 in, 1 out]
        n146 = property class="MB_Master"(reference=w312, error in=w313, "Properties:Slave ID"=w314) -> (reference out=w311:refnum<class "MB_Master.lvclass">, error out=w310:errorcluster)
        n147 = call <vilib>:"Read Holding Registers.vi"("error in (no error)"=w310, "quantity"=u16 40, "starting address"=u16 4224, "MB session in"=w311) -> ("error out"=w307:errorcluster, "Registers"=w308:u16[], "MB session out"=w318:refnum<class "MB_Master.lvclass">)  [unwired: 5 in]
        n148 = case shown="无错误" w307 {
          tunnel: w308 -> [w320 _]
          frame No Error {
            n149 = call "状态告警区.vi"("数组"=w320) -> ("状态告警区"=w319:T1)  [unwired: 10 in]
            "状态告警区" <- w319
            n150 = global write "VARCODMn全局变量.vi" "状态告警区"(w319) -> ()
            "状态告警区" <- w320
          }
          frame Error {
          }
        }
      }
      frame "读关键参数区" {
        n151 = Variant To Data(type=u8 1 ("Slave ID"), Variant=w325) -> (data=w323:u8)  [unwired: 1 in, 1 out]
        n152 = property class="MB_Master"(reference=w328, error in=w329, "Properties:Slave ID"=w323) -> (reference out=w327:refnum<class "MB_Master.lvclass">, error out=w326:errorcluster)
        n153 = call <vilib>:"Read Holding Registers.vi"("error in (no error)"=w326, "quantity"=u16 19, "starting address"=u16 4256, "MB session in"=w327) -> ("error out"=w321:errorcluster, "Registers"=w322:u16[], "MB session out"=w332:refnum<class "MB_Master.lvclass">)  [unwired: 5 in]
        n154 = case shown="无错误" w321 {
          tunnel: w322 -> [w334 _]
          frame No Error {
            n155 = call "关键参数区.vi"("数组"=w334) -> ("关键参数区"=w333:T3)  [unwired: 10 in]
            "关键参数区" <- w333
            n156 = global write "VARCODMn全局变量.vi" "关键参数区"(w333) -> ()
          }
          frame Error {
          }
        }
      }
      frame "读序列号" {
        n157 = Variant To Data(type=u8 1 ("Slave ID"), Variant=w340) -> (data=w338:u8)  [unwired: 1 in, 1 out]
        n158 = property class="MB_Master"(reference=w343, error in=w344, "Properties:Slave ID"=w338) -> (reference out=w342:refnum<class "MB_Master.lvclass">, error out=w341:errorcluster)
        n159 = call <vilib>:"Read Holding Registers.vi"("error in (no error)"=w341, "quantity"=u16 6, "starting address"=u16 4, "MB session in"=w342) -> ("error out"=w348:errorcluster, "Registers"=w337:u16[], "MB session out"=w347:refnum<class "MB_Master.lvclass">)  [unwired: 5 in]
        n160 = call "HexToString.vi"("数组"=w337) -> ("STRING"=w336:string[])  [unwired: 10 in]
        n161 = Index Array(array=w336) -> (element=w335:string)  [unwired: 1 in]
        "序列号" <- w335
        n162 = global write "VARCODMn全局变量.vi" "序列号"(w335) -> ()
      }
      frame "shutdown" {
        n163 = call-dynamic "Close Session.vi"("error in (no error)"=w351, "MB session in"=w349) -> ("error out"=w350:errorcluster)  [unwired: 9 in]
        n164 = Flush Queue(queue=w353) -> (queue out=w352:refnum<queue>)  [unwired: 1 in, 2 out]
        n165 = Release Queue(queue=w352) -> ()  [unwired: 2 in, 3 out]
      }
    }
    n166 = Unbundle By Name(w221) -> ("status"=w220:bool)
    n167 = Not(x=w220) -> (.not. x?=w219:bool)
    "status" <- w219
    n168 = global write "VARCODMn全局变量.vi" "通讯状态"(w219) -> ()
  }
  n169 = Release Queue(queue=w4, error in (no error)=w3) -> ()  [unwired: 1 in, 3 out]
